vi "ini_ini.vi"() -> ()   [LabVIEW 2023]
uses:
  <vilib>/Utility/config.llb/Write Key (String).vi
  <vilib>/Utility/config.llb/NI_LVConfig.lvlib
panel:
  out "配置文件路径":path
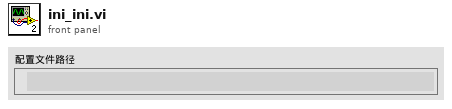
[diagram p1: front panel]
types:
  T1 = typedef "NI_LVConfig.lvlib/Config Data RefNum.ctl" = refnum<k1>
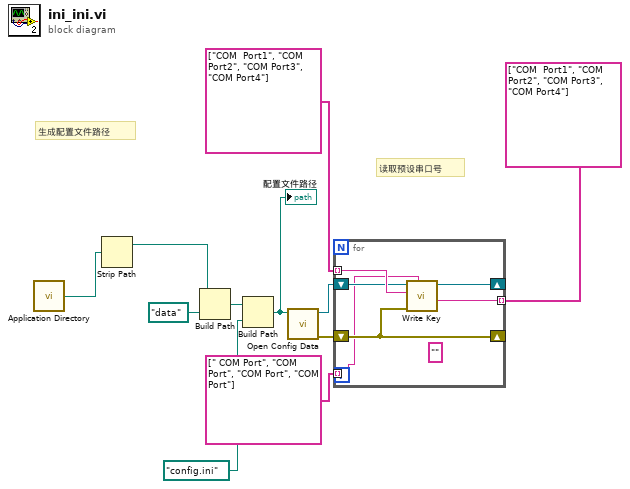
[diagram p0: block diagram]
diagram:
  # "读取预设串口号"
  # "生成配置文件路径"
  n1 = call <vilib>:"Application Directory.vi"() -> ("Application Directory"=w3:path)
  n2 = Strip Path(path=w3) -> (stripped path=w2:path)  [unwired: 1 out]
  n3 = Build Path(base path=w2, name or relative path=path "data" ("名称或相对路径")) -> (appended path=w11:path)
  n4 = Build Path(base path=w11, name or relative path=path "config.ini" ("名称或相对路径")) -> (appended path=w8:path)
  "配置文件路径" <- w8
  n5 = call <vilib>:"Open Config Data.vi"("configuration file path"=w8) -> ("error out"=w5:errorcluster, "refnum"=w6:T1)  [unwired: 8 in, 1 out]
  n6 = for {
    tunnel: string[] [" COM Port", "COM Port", "COM Port", "COM Port"] ("section") -> [w13] mode=indexing
    tunnel: string[] ["COM  Port1", "COM Port2", "COM Port3", "COM Port4"] ("section") -> [w16] mode=indexing
    shift-right: [w14] -> _
    shift-left: w6 -> [w15]
    shift-right: [w17] -> _
    shift-left: w5 -> [w17]
    tunnel: string[] ["COM  Port1", "COM Port2", "COM Port3", "COM Port4"] ("section") -> [w12] mode=indexing
    (unwired) "" ("section")
    n7 = call-poly <vilib>:"Write Key.vi"("section"=w13, "error in (no error)"=w17, "value"=w12, "key"=w16, "refnum"=w15) -> ("refnum out"=w14:T1)  [unwired: 4 in, 2 out]
  }
